vi "Get Reference.vi"(8 "error in (no error)":errorcluster, 11 "Class Reference Control in":refnum<class "Class Reference Control.lvclass">) -> (0 "error out":errorcluster, 2 "LabVIEW Class":refnum<vi>, 3 "Class Reference Control out":refnum<class "Class Reference Control.lvclass">)   [LabVIEW 2016, in "Class Reference Control.lvclass"]
uses:
  Class Reference Control.lvclass
  Class Reference Control.lvclass/Class Reference Control.ctl
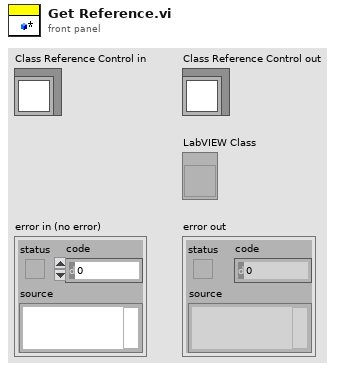
[diagram p1: front panel]
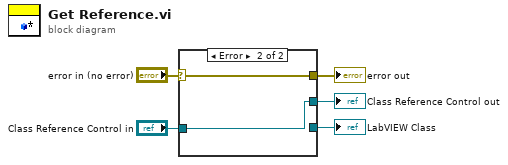
[diagram p0: block diagram]
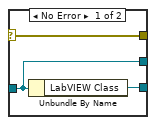
[diagram p2: hidden frame]
diagram:
  n1 = case shown="Error" "error in (no error)" {
    selector: "error in (no error)" -> [w8 w10]
    tunnel: [w8 w10] -> w4
    tunnel: [w7 w9] -> w2
    tunnel: "Class Reference Control in" -> [w7 w9]
    tunnel: [w6 _] -> w1
    frame No Error {
      n2 = Unbundle By Name(w7) -> ("LabVIEW Class"=w6:refnum<vi>)
    }
    frame Error {
    }
  }
  "error out" <- w4
  "Class Reference Control out" <- w2
  "LabVIEW Class" <- w1
